vi "Find Line.vi"(6 "Ignore Index? (D=-1)":i32=-1, 8 "Ignore line? (D=-1)":i32=-1, 9 "Z":dbl, 10 "X":dbl, 11 "All Lines":T1) -> (0 "Distance to nearest":dbl, 1 "Index on Line":i32, 2 "Nearest Line":i32, 3 "Line found?":bool)   [LabVIEW 2014]
uses:
  Libraries/Map Data Folder/All-Lines.ctl
  Libraries/Map Data Folder/LineCluster.ctl
  Libraries/Map Data Folder/LineConnection.ctl
  Libraries/Map Data Folder/Map Data.lvlib
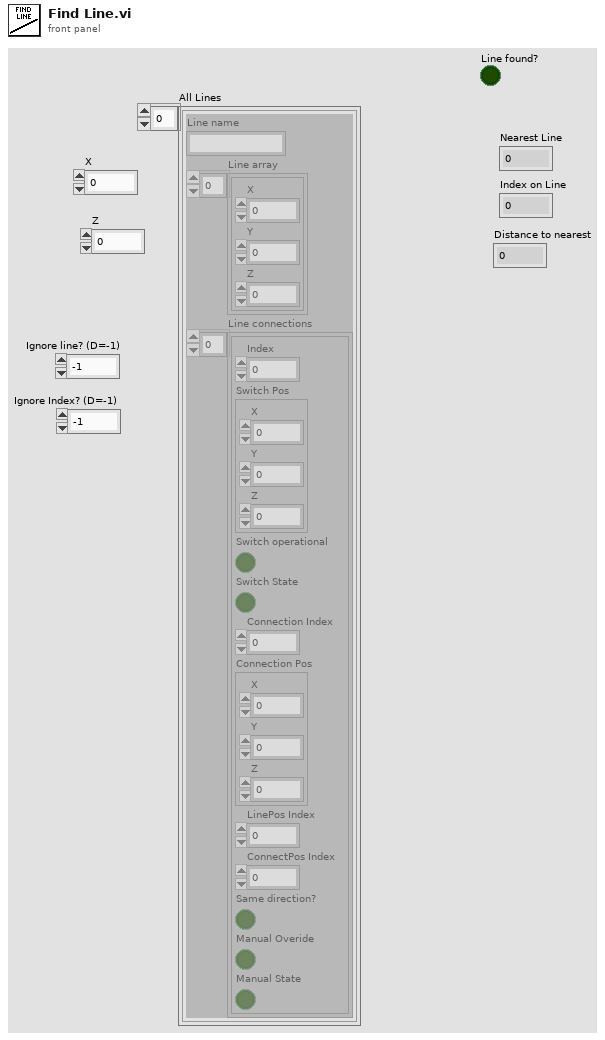
[diagram p1: front panel]
types:
  T1 = typedef "Map Data.lvlib/All-Lines.ctl" = T2[]
  T2 = typedef "Map Data.lvlib/LineCluster.ctl" = cluster{"Line name":string, "Line array":cluster{"X":dbl, "Y":dbl, "Z":dbl}[], "Line connections":T3[]}
  T3 = typedef "LineConnection.ctl" = cluster{"Index":i32, "Switch Pos":cluster{"X":dbl, "Y":dbl, "Z":dbl}, "Switch operational":bool, "Switch State":bool, "Connection Index":i32, "Connection Pos":cluster{"X":dbl, "Y":dbl, "Z":dbl}, "LinePos Index":i32, "ConnectPos Index":i32, "Same direction?":bool, "Manual Overide":bool, "Manual State":bool}
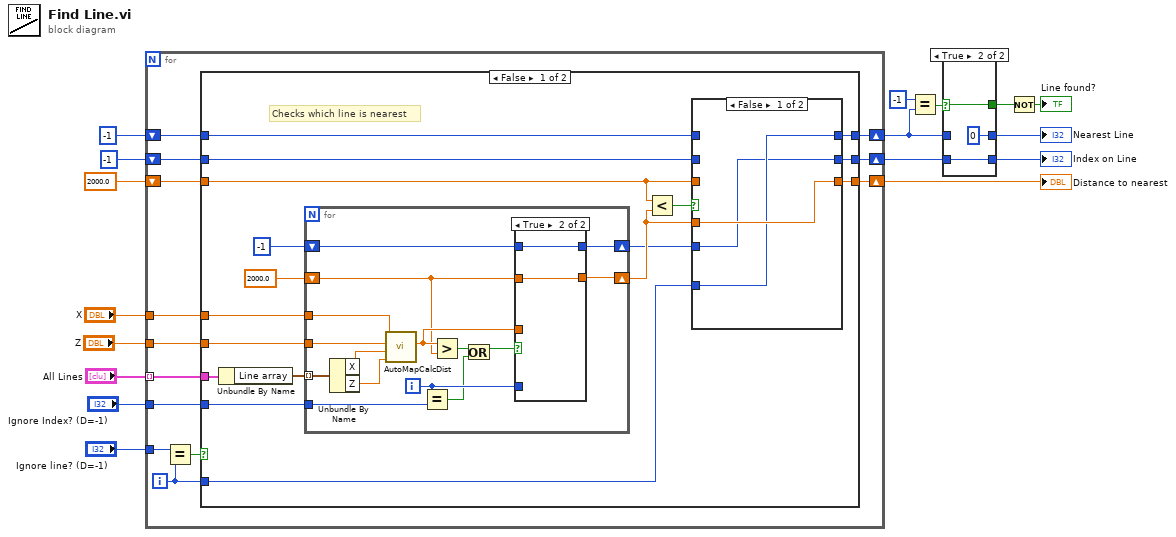
[diagram p0: block diagram]
diagram:
  n1 = for {
    tunnel: "All Lines" -> [w30] mode=indexing
    tunnel: "X" -> [w29]
    tunnel: "Z" -> [w28]
    shift-right: [w27] -> w15
    shift-left: 2000.0 ("Distance") -> [w24]
    shift-right: [w26] -> w3
    shift-left: -1 -> [w25]
    shift-right: [w22] -> w2
    shift-left: -1 -> [w23]
    tunnel: "Ignore line? (D=-1)" -> [w20]
    tunnel: "Ignore Index? (D=-1)" -> [w18]
    i -> [w21]
    n2 = Equal?(x=w20, y=w21) -> (x = y?=w19:bool)
    n3 = case shown="False" w19 {
      tunnel: w30 -> [w47 _]
      tunnel: w29 -> [w45 _]
      tunnel: w28 -> [w44 _]
      tunnel: [w42 w74] -> w27
      tunnel: [w41 w73] -> w26
      tunnel: w25 -> [w40 w73]
      tunnel: w24 -> [w39 w74]
      tunnel: w23 -> [w36 w75]
      tunnel: [w33 w75] -> w22
      tunnel: w21 -> [w32 _]
      tunnel: w18 -> [w31 _]
      frame False {
        # "Checks which line is nearest"
        n4 = Unbundle By Name(w47) -> ("Line array"=w46:cluster{"X":dbl, "Y":dbl, "Z":dbl}[])
        n5 = for {
          tunnel: w45 -> [w68]
          tunnel: w46 -> [w67] mode=indexing
          tunnel: w44 -> [w63]
          shift-right: [w60] -> w38
          shift-left: 2000.0 ("Distance") -> [w61]
          shift-right: [w58] -> w34
          shift-left: -1 -> [w59]
          tunnel: w31 -> [w56]
          i -> [w57]
          n6 = Unbundle By Name(w67) -> ("X"=w64:dbl, "Z"=w65:dbl)
          n7 = call "AutoMapCalcDist.vi"("Y2"=w65, "X2"=w64, "Y1"=w63, "X1"=w68) -> ("Distance"=w62:dbl)  [unwired: 7 in]
          n8 = Equal?(x=w57, y=w56) -> (x = y?=w54:bool)
          n9 = Greater?(x=w62, y=w61) -> (0:w66:bool)
          n10 = Or(x=w66, y=w54) -> (x .or. y?=w55:bool)
          n11 = case shown="True" w55 {
            tunnel: w62 -> [w70 _]
            tunnel: [w70 w72] -> w60
            tunnel: w61 -> [_ w72]
            tunnel: w59 -> [_ w71]
            tunnel: w57 -> [w69 _]
            tunnel: [w69 w71] -> w58
            frame False {
            }
            frame True {
            }
          }
        }
        n12 = Less?(x=w39, y=w38) -> (x < y?=w37:bool)
        n13 = case shown="False" w37 {
          tunnel: w38 -> [w50 _]
          tunnel: [w50 w52] -> w42
          tunnel: w39 -> [_ w52]
          tunnel: w32 -> [w49 _]
          tunnel: [w49 w53] -> w41
          tunnel: w40 -> [_ w53]
          tunnel: w36 -> [_ w51]
          tunnel: w34 -> [w48 _]
          tunnel: [w48 w51] -> w33
          frame False {
          }
          frame True {
          }
        }
      }
      frame True {
      }
    }
  }
  "Distance to nearest" <- w15
  n14 = Equal?(x=-1, y=w3) -> (x = y?=w5:bool)
  n15 = case shown="True" w5 {
    selector: w5 -> [w76 w81]
    tunnel: [w76 w81] -> w6
    tunnel: w3 -> [w78 _]
    tunnel: [w78 0] -> w4
    tunnel: w2 -> [w77 w80]
    tunnel: [w77 w80] -> w1
    frame False {
    }
    frame True {
    }
  }
  "Nearest Line" <- w4
  "Index on Line" <- w1
  n16 = Not(x=w6) -> (.not. x?=→"Line found?":bool)
